vi "Test Command WPIN Response.vi"(8 "error in (no error)":errorcluster, 11 "TestCase in":refnum<class "Test ADC Command.lvclass">) -> (0 "error out":errorcluster, 3 "TestCase out":refnum<class "Test ADC Command.lvclass">)   [LabVIEW 2019, in "Test ADC Command.lvclass"]
uses:
  Test ADC Command.lvclass
  SIMULATED/SIMULATED.lvclass
  <vilib>/addons/_JKI Toolkits/VI Tester/TestCase.llb/TestCase.lvclass
  Serial Devices.lvclass
  C:/Program Files (x86)/National Instruments/LabVIEW 2019/vi.lib/addons/_JKI Toolkits/VI Tester/TestCase.llb/TestCase.lvclass
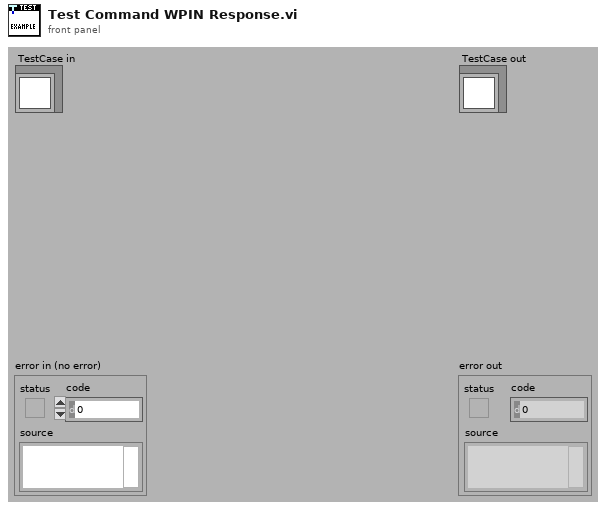
[diagram p1: front panel]
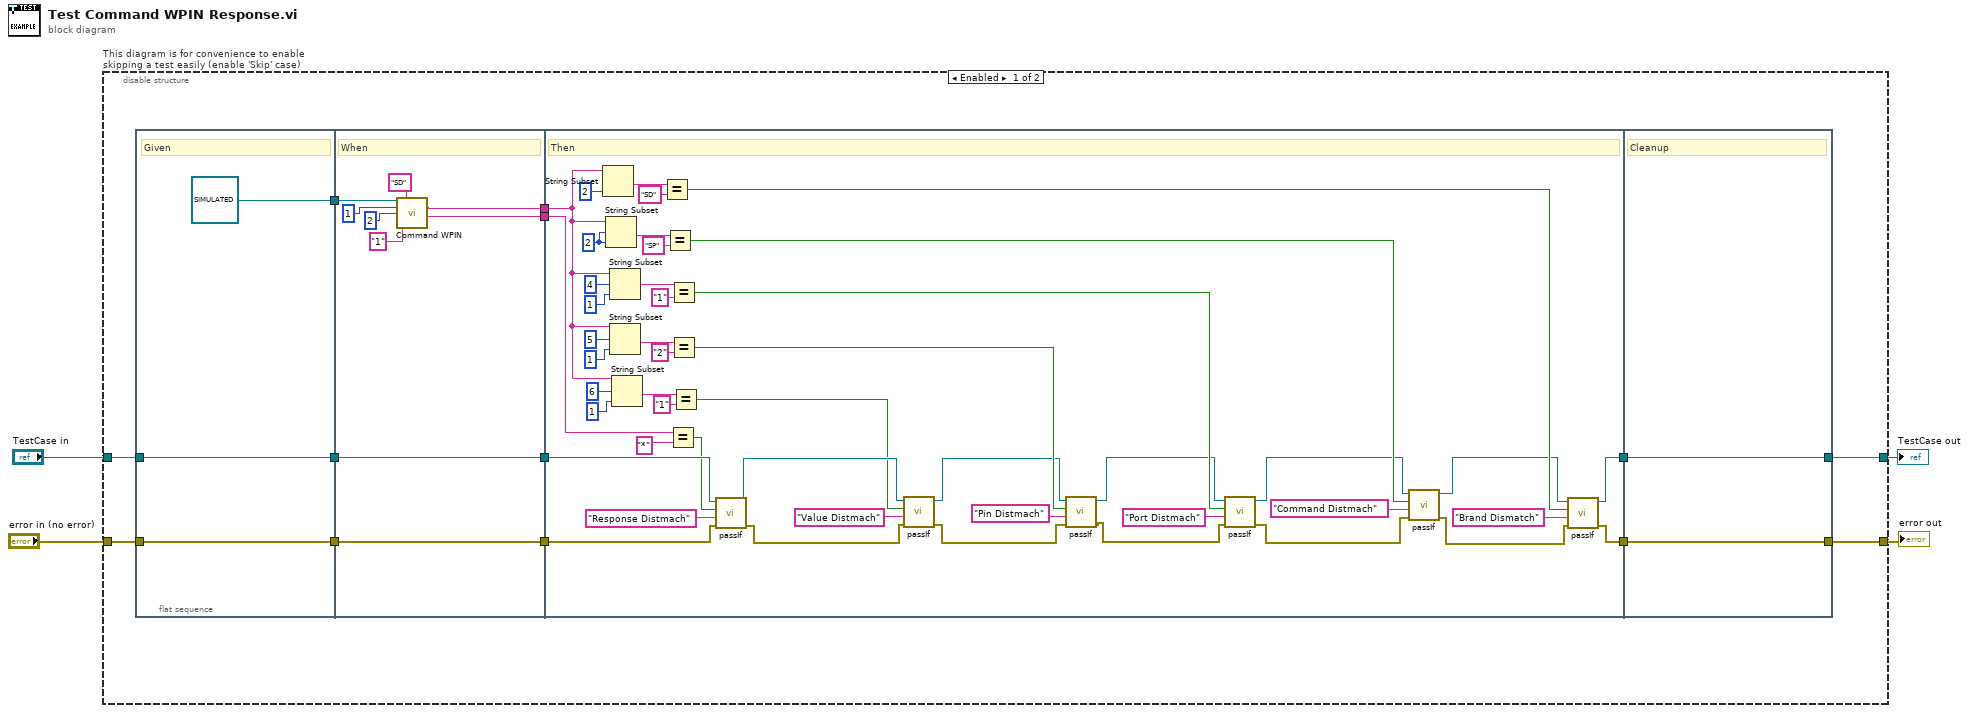
[diagram p0: block diagram]
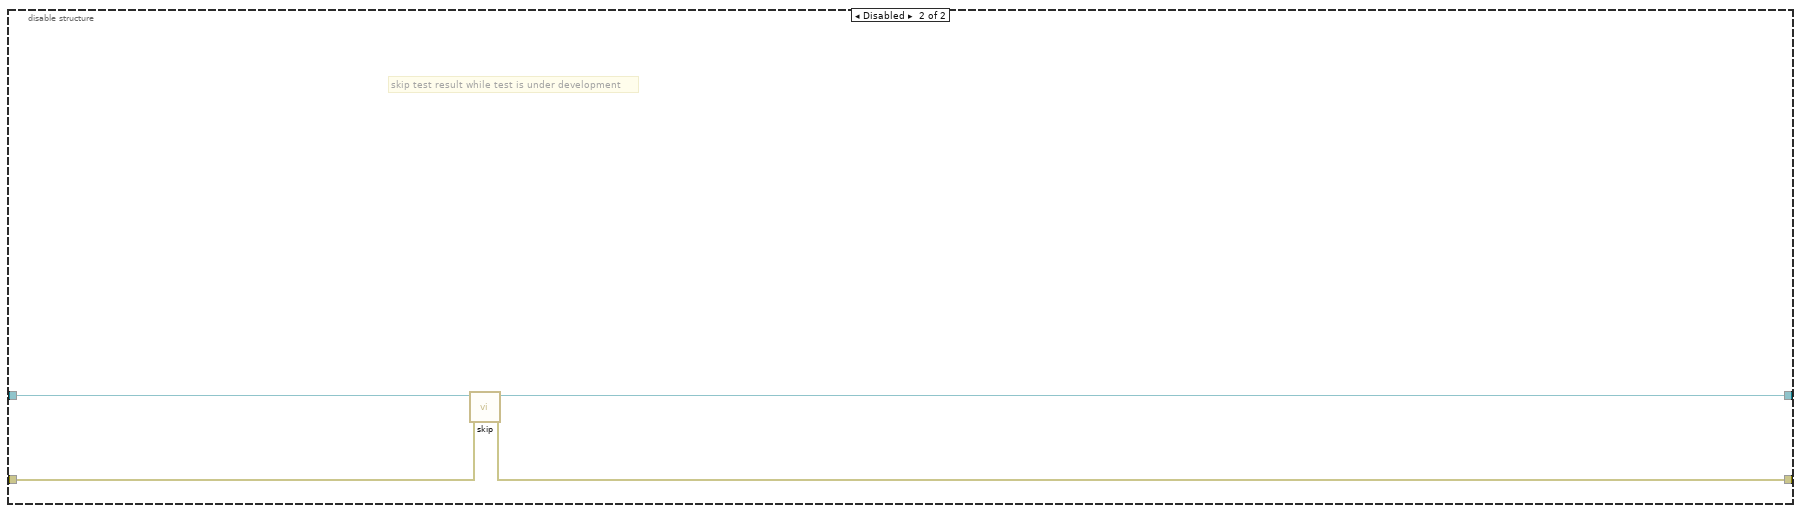
[diagram p2: hidden frame]
diagram:
  n1 = disable-structure "This diagram is for convenience to enable skipping a test easily (enable 'Skip' case)" shown="Enabled" {
    disable-tunnel: "TestCase in" -> [w16 w82]
    disable-tunnel: [w9 w80] -> w3
    disable-tunnel: [w8 w81] -> w4
    disable-tunnel: "error in (no error)" -> [w13 w79]
    frame Enabled {
      n2 = flat-sequence {
        tunnel: [w20] -> w17
        tunnel: w16 -> [w20]
        tunnel: [w19] -> w14
        tunnel: w13 -> [w19]
        tunnel: [refnum<class "SIMULATED.lvclass"> refnum ("SIMULATED.lvclass")] -> w7
        tunnel: w17 -> [w28]
        tunnel: [w28] -> w15
        tunnel: w14 -> [w29]
        tunnel: [w29] -> w12
        tunnel: w7 -> [w27]
        tunnel: [w21] -> w6
        tunnel: [w22] -> w5
        tunnel: w15 -> [w52]
        tunnel: w12 -> [w51]
        tunnel: [w71] -> w11
        tunnel: [w72] -> w10
        tunnel: w6 -> [w36]
        tunnel: w5 -> [w55]
        tunnel: [w78] -> w9
        tunnel: w11 -> [w78]
        tunnel: [w77] -> w8
        tunnel: w10 -> [w77]
        frame #0 {
          # "Given"
        }
        frame #1 {
          # "When"
          n3 = call "Command WPIN.vi"("Serial Devices in"=w27, "Device"="SD", "Puerto"=u8 1 ("Chanel"), "Pin"=u8 2, "Valor"="1") -> ("Command"=w21:string, "Expected"=w22:string)  [unwired: 7 in, 2 out]
        }
        frame #2 {
          w67 = 2 ("offset (0)")
          # "Then"
          n4 = String Subset(string=w36, length (rest)=2 ("offset (0)")) -> (substring=w75:string)  [unwired: 1 in]
          n5 = String Subset(string=w36, offset (0)=w67, length (rest)=w67) -> (substring=w68:string)
          n6 = String Subset(string=w36, offset (0)=4, length (rest)=1 ("length (rest)")) -> (substring=w45:string)
          n7 = String Subset(string=w36, offset (0)=5, length (rest)=1 ("length (rest)")) -> (substring=w47:string)
          n8 = String Subset(string=w36, offset (0)=6, length (rest)=1 ("length (rest)")) -> (substring=w39:string)
          n9 = Equal?(x=w75, y="SD") -> (x = y?=w73:bool)
          n10 = Equal?(x=w68, y="SP") -> (x = y?=w65:bool)
          n11 = Equal?(x=w55, y="*") -> (x = y?=w50:bool)
          n12 = Equal?(x=w45, y="1") -> (x = y?=w56:bool)
          n13 = Equal?(x=w47, y="2") -> (x = y?=w41:bool)
          n14 = Equal?(x=w39, y="1") -> (x = y?=w30:bool)
          n15 = call-dynamic "passIf.vi"("error in (no error)"=w51, "message (\"\")"="Response Distmach" ("message (\"\")"), "pass"=w50, "TestCase in"=w52) -> ("error out"=w34:errorcluster, "TestCase out"=w32:refnum<class "Test ADC Command.lvclass">)  [unwired: 6 in]
          n16 = call-dynamic "passIf.vi"("error in (no error)"=w34, "message (\"\")"="Value Distmach" ("message (\"\")"), "pass"=w30, "TestCase in"=w32) -> ("error out"=w33:errorcluster, "TestCase out"=w31:refnum<class "Test ADC Command.lvclass">)  [unwired: 6 in]
          n17 = call-dynamic "passIf.vi"("error in (no error)"=w33, "message (\"\")"="Pin Distmach" ("message (\"\")"), "pass"=w41, "TestCase in"=w31) -> ("error out"=w42:errorcluster, "TestCase out"=w43:refnum<class "Test ADC Command.lvclass">)  [unwired: 6 in]
          n18 = call-dynamic "passIf.vi"("error in (no error)"=w42, "message (\"\")"="Port Distmach" ("message (\"\")"), "pass"=w56, "TestCase in"=w43) -> ("error out"=w61:errorcluster, "TestCase out"=w63:refnum<class "Test ADC Command.lvclass">)  [unwired: 6 in]
          n19 = call-dynamic "passIf.vi"("error in (no error)"=w61, "message (\"\")"="Command Distmach" ("message (\"\")"), "pass"=w65, "TestCase in"=w63) -> ("error out"=w60:errorcluster, "TestCase out"=w66:refnum<class "Test ADC Command.lvclass">)  [unwired: 6 in]
          n20 = call-dynamic "passIf.vi"("error in (no error)"=w60, "message (\"\")"="Brand Dismatch" ("message (\"\")"), "pass"=w73, "TestCase in"=w66) -> ("error out"=w72:errorcluster, "TestCase out"=w71:refnum<class "Test ADC Command.lvclass">)  [unwired: 6 in]
        }
        frame #3 {
          # "Cleanup"
        }
      }
    }
    frame Disabled {
      # "skip test result while test is under development"
      n21 = call <vilib>:"skip.vi"("error in (no error)"=w79, "TestCase in"=w82) -> ("error out"=w81:errorcluster, "TestCase out"=w80:refnum<class "Test ADC Command.lvclass">)  [unwired: 8 in]
    }
  }
  "error out" <- w4
  "TestCase out" <- w3
